vi "Run Trivial vi on server.vi"() -> ()   [LabVIEW 2022 SP3]
panel:
  out "Loop Number":i32
  out "Difference":dbl
  out "Server time":dbl
  in  "trivial.vi type":refnum<vi>
  out "Loop comms":errorcluster
  in  "stop":bool
  out "Vi Reference":errorcluster
  out "Application reference":errorcluster
  in  "IP Number":string="131.227.181.40"
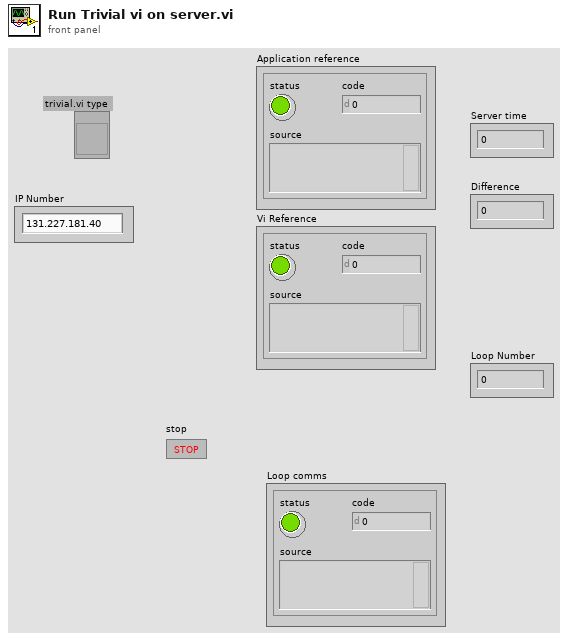
[diagram p1: front panel]
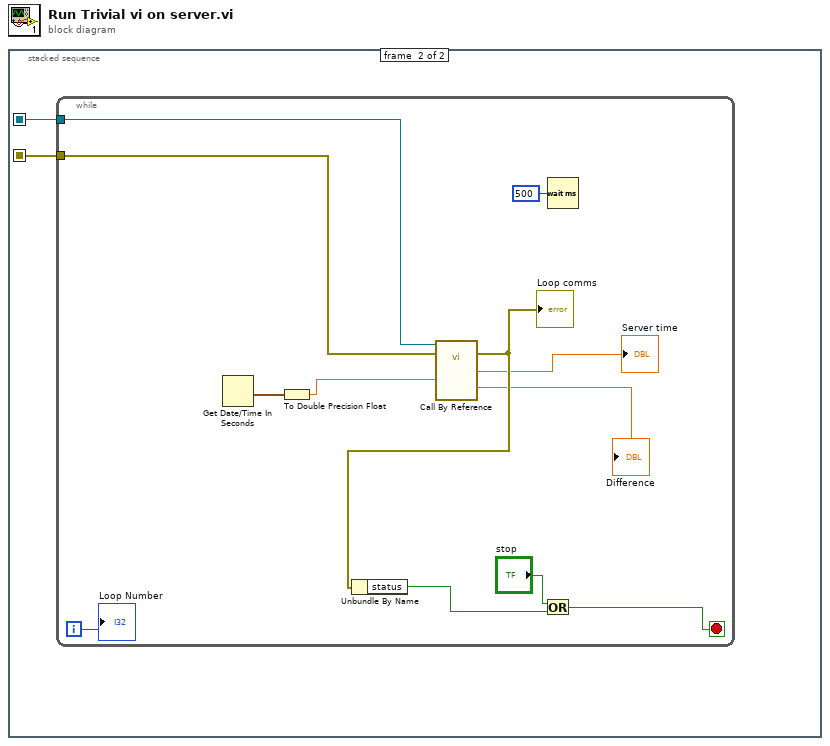
[diagram p0: block diagram]
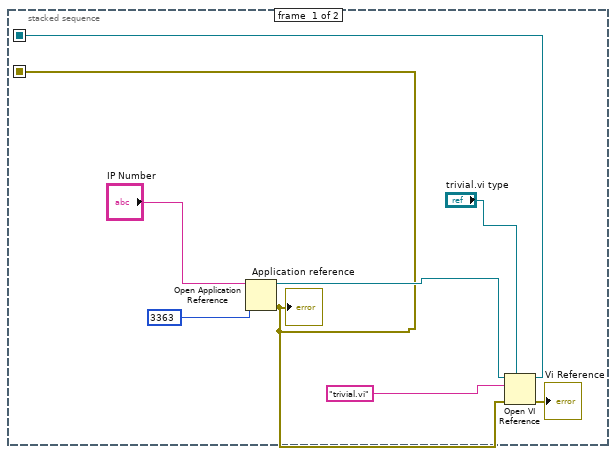
[diagram p2: hidden frame]
diagram:
  n1 = stacked-sequence {
    seq-local: [w2 _] -> [_ w10]
    seq-local: [w4 _] -> [_ w9]
    frame #0 {
      n2 = Open Application Reference(10:u16 3363 ("port number or service name (3363)"), 11:"IP Number") -> (0:w4:errorcluster, 3:w5:refnum<vi>)  [unwired: 1 in, 1 out]
      "Application reference" <- w4
      n3 = Open VI Reference(type specifier VI Refnum (for type only)="trivial.vi type", application reference (local)=w5, vi path="trivial.vi", error in (no error)=w4) -> (vi reference=w2:refnum<vi>, error out=→"Vi Reference":errorcluster)  [unwired: 2 out]
    }
    frame #1 {
      n4 = while {
        tunnel: w10 -> [w21]
        tunnel: w9 -> [w20]
        i -> [w11]
        stop <- w16 stop-if-true
        n5 = Get Date/Time In Seconds() -> (seconds since 1Jan1904=w15:timestamp)
        n6 = To Double Precision Float(number=w15) -> (double precision float=w14:dbl)
        n7 = call-by-ref "Call By Reference"(reference=w21, error in=w20, "Client time"=w14) -> (error out=w19:errorcluster, "Server time"=→"Server time":dbl, "Difference"=→"Difference":dbl)  [unwired: 1 out]
        "Loop comms" <- w19
        n8 = Unbundle By Name(w19) -> ("status"=w17:bool)
        n9 = Or(x="stop", y=w17) -> (x .or. y?=w16:bool)
        n10 = Wait (ms)(milliseconds to wait=u32 500) -> ()  [unwired: 1 out]
        "Loop Number" <- w11
      }
    }
  }
